vi "Write Scale Marker FG Color.vi"(8 "error in (no error)":errorcluster, 9 "Index":i32, 10 "Marker FG Color":u32(colorbox), 11 "2D Plot.lvclass in":refnum<class "2D Plot.lvclass">) -> (0 "error out":errorcluster, 3 "2D Plot.lvclass out":refnum<class "2D Plot.lvclass">)   [LabVIEW 2020, in "2D Plot.lvclass"]
uses:
  <vilib>/Math Plots/2D Math Plots/2D Plot/2D Plot/2D Plot.lvclass
  <vilib>/Math Plots/2D Math Plots/2D Plot/2D Plot/2D Plot.lvclass/2D Plot.ctl
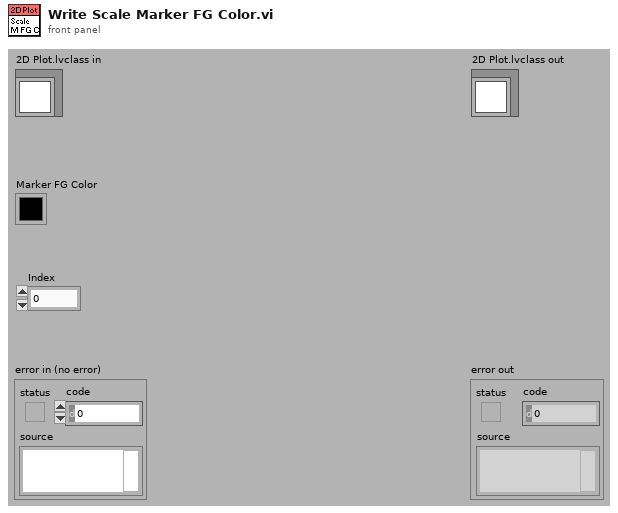
[diagram p1: front panel]
types:
  T1 = typedef "2D Plot.lvclass/Scale Array.ctl" = T2[]
  T2 = typedef "2D Plot.lvclass/Scale Cluster.ctl" = cluster{"General":cluster{"Editable":bool, "Flipped":bool, "Mapping Mode":u8, "Visible":bool, "Style":u8, "Scale Fit":u8}, "Offset and Multiplier":T3, "Range":cluster{"Minimum":dbl, "Maximum":dbl, "Increment":dbl, "Minor Increment":dbl, "Start":dbl}, "Tick Color":cluster{"Major Color":u32, "Minor Color":u32}, "Gird Color":cluster{"Major Color":u32, "Minor Color":u32}, "Marker":cluster{"Visible":bool, "FG Color":u32, "BG Color":u32, "Font Name":string, "Font Size":u32, "Font Bold":bool, "Font Italic":bool, "Font Strikeout":bool, "Font Underline":bool}, "Name Label":cluster{"Visible":bool, "FG Color":u32, "BG Color":u32, "Font Name":string, "Font Size":u32, "Font Bold":bool, "Font Italic":bool, "Font Strikeout":bool, "Font Underline":bool, "Justification":enum16{"Left", "Center", "Right"}, "Text":string}}
  T3 = typedef "LVOffsetAndMultiplierTypeDef.ctl" = cluster{"Offset":dbl, "Multiplier":dbl}
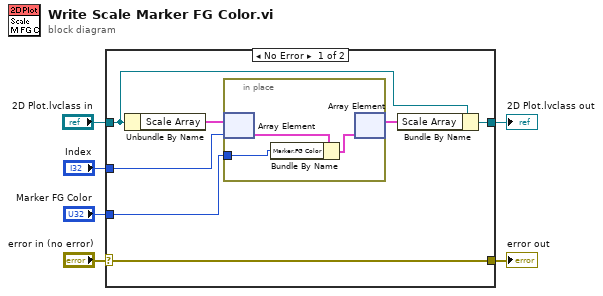
[diagram p0: block diagram]
diagram:
  n1 = case shown="No Error" "error in (no error)" {
    selector: "error in (no error)" -> [w13 w17]
    tunnel: "Marker FG Color" -> [w9 _]
    tunnel: "2D Plot.lvclass in" -> [w12 w18]
    tunnel: [w11 w18] -> w5
    tunnel: [w13 w17] -> w3
    tunnel: "Index" -> [w7 _]
    frame No Error {
      n2 = Unbundle By Name(w12) -> ("Scale Array"=w10:T1)
      n3 = in-place {
        in-place-border: w9 -> [w15]
        n4 = in-place-array #1(w10, w7) -> (w16:T2)
        n5 = Bundle By Name(cluster=w16, "Marker.FG Color"=w15) -> (w14:T2)
        n6 = in-place-array #1(w14) -> (w8:T1)  [unwired: 1 out]
      }
      n7 = Bundle By Name(cluster=w12, "Scale Array"=w8) -> (w11:refnum<class "2D Plot.lvclass">)
    }
    frame Error {
    }
  }
  "error out" <- w3
  "2D Plot.lvclass out" <- w5
